vi "movera.vi"(2 "SetPosition":sgl format="%.2f", 3 "EXP300 Axis":i8=1, 4 "ESP300 Add.":i32=3) -> ()   [LabVIEW 2010]
panel:
  out "Current Position":dbl
  out "Time to wait (s)":i16
  # "Stage Moving"
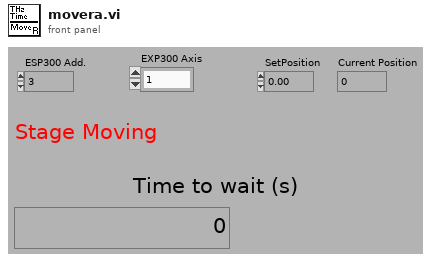
[diagram p1: front panel]
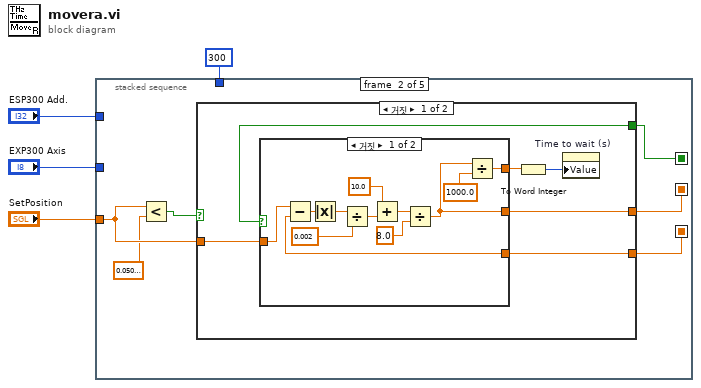
[diagram p0: block diagram]
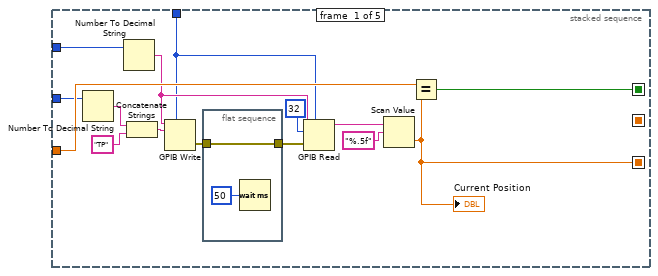
[diagram p2: hidden frame]
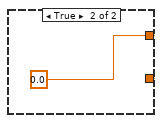
[diagram p3: hidden frame]
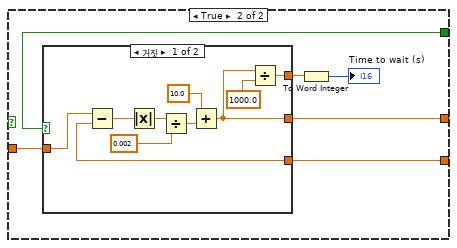
[diagram p4: hidden frame]
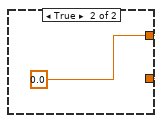
[diagram p5: hidden frame]
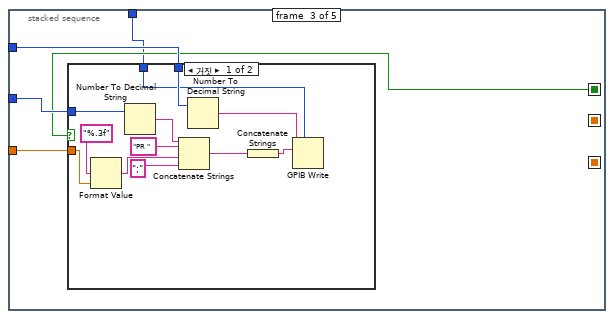
[diagram p6: hidden frame]
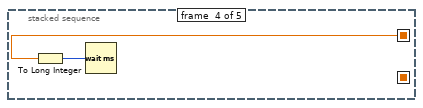
[diagram p8: hidden frame]
diagram:
  n1 = stacked-sequence {
    seq-local: [w18 _ _ _ _] -> [_ w27 _ _ _]
    seq-local: [w16 _ _ _ _] -> [_ w26 w65 _ _]
    seq-local: [_ w25 _ _ _] -> [_ _ _ w82 _]
    tunnel: "ESP300 Add." -> [w15 _ w68 _ _]
    tunnel: "EXP300 Axis" -> [w11 _ w67 _ _]
    tunnel: "SetPosition" -> [w17 w23 w66 _ _]
    tunnel: 300 ("timeout ms (488.2 global)") -> [w9 _ w64 _ _]
    frame #0 {
      n2 = Number To Decimal String(number=w11) -> (decimal integer string=w7:string)  [unwired: 1 in]
      n3 = Number To Decimal String(number=w15) -> (decimal integer string=w13:string)  [unwired: 1 in]
      n4 = Concatenate Strings(w7, "TP" ("string")) -> (w10:string)
      n5 = GPIB Write(0:w13, 1:w10, 4:w9) -> (6:w6:errorcluster)  [unwired: 2 in, 1 out]
      n6 = flat-sequence {
        tunnel: w6 -> [w21]
        tunnel: [w21] -> w5
        frame #0 {
          n7 = Wait (ms)(milliseconds to wait=u32 50) -> ()  [unwired: 1 out]
        }
      }
      n8 = GPIB Read(0:w13, 1:32 ("byte count"), 3:w5, 4:w9) -> (5:w14:string)  [unwired: 1 in, 2 out]
      n9 = Scan Value(string=w14, format string="%.5f") -> (value=w18:dbl)  [unwired: 1 in, 1 out]
      "Current Position" <- w18
      n10 = Equal?(x=w17, y=w18) -> (x = y?=w16:bool)
    }
    frame #1 {
      n11 = Less?(x=w23, y=sgl 0.05) -> (x < y?=w24:bool)
      n12 = case shown="거짓" w24 {
        tunnel: w23 -> [w31 w52]
        tunnel: w27 -> [w30 w51]
        tunnel: w26 -> [w32 w50]
        tunnel: [w29 w49] -> w25
        frame False {
          n13 = case shown="거짓" w32 {
            tunnel: w31 -> [w42 _]
            tunnel: w30 -> [w41 _]
            tunnel: [w37 w46] -> w33
            tunnel: [w35 w46] -> w29
            frame False {
              n14 = Subtract(x=w42, y=w41) -> (x-y=w43:dbl)
              n15 = Absolute Value(x=w43) -> (abs(x)=w44:dbl)
              n16 = Divide(x=w44, y=0.002) -> (x/y=w40:dbl)
              n17 = Add(x=10.0, y=w40) -> (x+y=w36:dbl)
              n18 = Divide(x=w36, y=8.0) -> (x/y=w35:dbl)
              n19 = Divide(x=w35, y=1000.0) -> (x/y=w37:dbl)
            }
            frame True {
              w46 = 0.0
            }
          }
          n20 = To Word Integer(number=w33) -> (16bit integer=w28:i16)
          n21 = property on="Time to wait (s)" class="DigNum (엄격한)"("Value"=w28) -> ()  [unwired: 2 in, 2 out]
        }
        frame True {
          n22 = case shown="거짓" w50 {
            tunnel: w52 -> [w59 _]
            tunnel: w51 -> [w58 _]
            tunnel: [w54 w63] -> w48
            tunnel: [w53 w63] -> w49
            frame False {
              n23 = Subtract(x=w59, y=w58) -> (x-y=w60:dbl)
              n24 = Absolute Value(x=w60) -> (abs(x)=w61:dbl)
              n25 = Divide(x=w61, y=0.002) -> (x/y=w57:dbl)
              n26 = Add(x=10.0, y=w57) -> (x+y=w53:dbl)
              n27 = Divide(x=w53, y=1000.0) -> (x/y=w54:dbl)
            }
            frame True {
              w63 = 0.0
            }
          }
          n28 = To Word Integer(number=w48) -> (16bit integer=→"Time to wait (s)":i16)
        }
      }
    }
    frame #2 {
      n29 = case shown="거짓" w65 {
        tunnel: w68 -> [w80 _]
        tunnel: w67 -> [w78 _]
        tunnel: w66 -> [w76 _]
        tunnel: w64 -> [w73 _]
        frame False {
          n30 = Format Value(format string="%.3f", value (0)=w76) -> (output string=w75:string)  [unwired: 1 in]
          n31 = Number To Decimal String(number=w78) -> (decimal integer string=w71:string)  [unwired: 1 in]
          n32 = Concatenate Strings(w71, "PR " ("string"), w75, ";" ("string")) -> (w70:string)
          n33 = Number To Decimal String(number=w80) -> (decimal integer string=w79:string)  [unwired: 1 in]
          n34 = Concatenate Strings(w70) -> (w69:string)
          n35 = GPIB Write(0:w79, 1:w69, 4:w73) -> ()  [unwired: 2 in, 2 out]
        }
        frame True {
        }
      }
    }
    frame #3 {
      n36 = To Long Integer(number=w82) -> (32bit integer=w81:i32)
      n37 = Wait (ms)(milliseconds to wait=w81) -> ()  [unwired: 1 out]
    }
    frame #4 {
    }
  }
